vi "SolveIntersectionStrip.vi"(7 "ct":dbl=10.0 format="%.2f", 8 "Root method":bool, 10 "strip":cluster{"radius":dbl, "h":dbl, "w":dbl}={"radius"=10.0, "h"=5.0, "w"=4.0} {"radius" format="%.2f"; "w" format="%.2f"; "h" format="%.2f"}, 11 "P":cluster{"x":dbl, "y":dbl, "z":dbl}={"x"=-4.0, "y"=0.0, "z"=4.0} {"x" format="%.2f"; "z" format="%.2f"; "y" format="%.2f"}) -> (0 "XY Graph":T1(graph), 1 "Array":dbl[][](array[numeric]) format="%.2f", 2 "sigma":dbl=4.0 format="%.2f", 3 "d":dbl=4.0 format="%.2f")   [LabVIEW 2022 SP3]
uses:
  <vilib>/gmath/NI_Gmath.lvlib
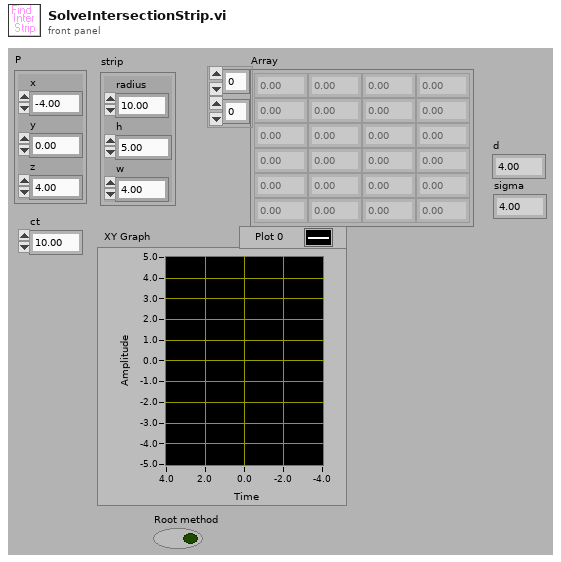
[diagram p1: front panel]
types:
  T1 = cluster{"Array Constant":dbl[], "Array Constant":dbl[]}[]
  T2 = cluster{"x,y,z[0]":dbl, "x,y,z[1]":dbl, "x,y,z[2]":dbl}
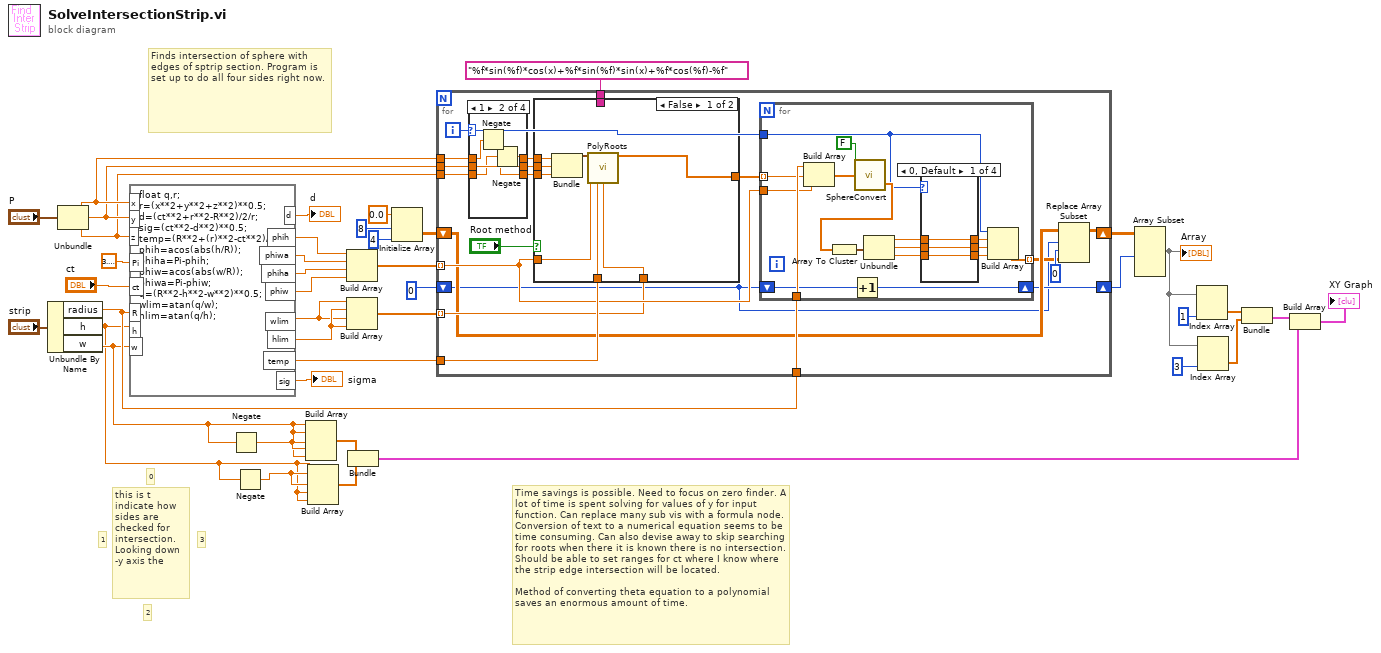
[diagram p0: block diagram]
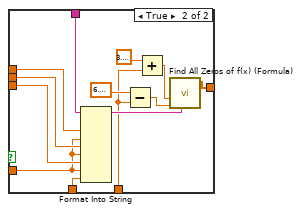
[diagram p2: hidden frame]
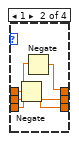
[diagram p3: hidden frame]
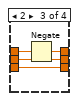
[diagram p4: hidden frame]
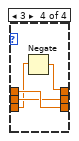
[diagram p5: hidden frame]
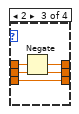
[diagram p7: hidden frame]
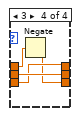
[diagram p8: hidden frame]
diagram:
  # "Finds intersection of sphere with edges of sptrip section. Program is set up to do all four sides right now."
  # "Time savings is possible. Need to focus on zero finder. A lot of time is spent solving for values of y for input function. Can replace many sub vis with a formula node. Conversion of text to a numerical equation seems to be time consuming. Can also devise away to skip searching for roots when there it is known there is no intersection. Should be able to set ranges for ct where I know where the strip edge intersection will be located.\n\nMethod of converting theta equation to a polynomial saves an enormous amount of time."
  # "3"
  # "2"
  # "1"
  # "0"
  # "this is t indicate how  sides are checked for intersection. Looking down -y axis the"
  n1 = Unbundle By Name("strip") -> ("radius"=w34:dbl, "h"=w13:dbl, "w"=w14:dbl)
  n2 = Unbundle("P") -> ("x"=w7:dbl, "y"=w6:dbl, "z"=w5:dbl)
  n3 = formula code="float q,r;\nr=(x**2+y**2+z**2)**0.5;\nd=(ct**2+r**2-R**2)/2/r;\nsig=(ct**2-d**2)**0.5;\ntemp=(R**2+(r)**2-ct**2)/2/R;\nphih=acos(abs(h/R));\nphiha=Pi-phih;\nphiw=acos(abs(w/R));\nphiwa=Pi-phiw;\nq=(R**2-h**2-w**2)**0.5;\nwlim=atan(q/w);\nhlim=atan(q/h);"("x"=w7, "y"=w6, "z"=w5, "ct"="ct", "R"=w34, "h"=w13, "w"=w14, "Pi"=3.141592653589793) -> ("d"=→"d":dbl, "sig"=→"sigma":dbl, "temp"=w38:dbl, "phih"=w28:dbl, "phiw"=w27:dbl, "phiha"=w31:dbl, "phiwa"=w32:dbl, "hlim"=w26:dbl, "wlim"=w25:dbl)
  n4 = Negate(x=w14) -> (-x=w20:dbl)
  n5 = Negate(x=w13) -> (-x=w19:dbl)
  n6 = Build Array(w14, w14, w20, w20, w14) -> (w18:dbl[])
  n7 = Build Array(w13, w19, w19, w13, w13) -> (w17:dbl[])
  n8 = Build Array(w28, w32, w31, w27) -> (w36:dbl[])
  n9 = Build Array(w25, w26, w25, w26) -> (w30:dbl[])
  n10 = Bundle(w18, w17) -> (w15:cluster{dbl[], dbl[]})  [unwired: 1 out]
  n11 = Initialize Array(0.0, 8, 4) -> (w11:dbl[][])
  n12 = for {
    tunnel: w38 -> [w61]
    tunnel: "%f*sin(%f)*cos(x)+%f*sin(%f)*sin(x)+%f*cos(%f)-%f" ("formula") -> [w57]
    tunnel: w36 -> [w55] mode=indexing
    tunnel: w34 -> [w54]
    shift-right: [w51] -> w10
    shift-left: w11 -> [w46]
    tunnel: w30 -> [w53] mode=indexing
    shift-right: [w44] -> w8
    shift-left: 0 -> [w43]
    tunnel: w7 -> [w49]
    tunnel: w6 -> [w48]
    tunnel: w5 -> [w47]
    i -> [w56]
    n13 = case shown="1" w56 {
      tunnel: [w118 w119 w124 w130] -> w60
      tunnel: w49 -> [w118 w121 w127 w129]
      tunnel: [w117 w123 w126 w131] -> w59
      tunnel: w48 -> [w117 w123 w126 w131]
      tunnel: [w116 w120 w125 w128] -> w58
      tunnel: w47 -> [w116 w122 w125 w130]
      frame 0, Default {
      }
      frame 1 {
        n14 = Negate(x=w121) -> (-x=w120:dbl)
        n15 = Negate(x=w122) -> (-x=w119:dbl)
      }
      frame 2 {
        n16 = Negate(x=w127) -> (-x=w124:dbl)
      }
      frame 3 {
        n17 = Negate(x=w129) -> (-x=w128:dbl)
      }
    }
    n18 = case shown="False" "Root method" {
      tunnel: w61 -> [w66 w82]
      tunnel: w60 -> [w65 w81]
      tunnel: w59 -> [w64 w80]
      tunnel: w58 -> [w63 w79]
      tunnel: w57 -> [_ w78]
      tunnel: w55 -> [w69 w77]
      tunnel: w53 -> [w67 w71]
      tunnel: [w68 w70] -> w52
      frame False {
        n19 = Bundle("z"=w65, "y"=w64, "z"=w63) -> (w62:cluster{"z":dbl, "y":dbl, "z":dbl})  [unwired: 1 out]
        n20 = call "PolyRoots.vi"("P"=w62, "phi"=w69, "constant"=w66, "theta lim"=w67) -> ("Polynomial Roots"=w68:dbl[])  [unwired: 2 in, 9 out]
      }
      frame True {
        n21 = Format Into String(format string=w78, w81, w77, w80, w77, w79, w77, w82) -> (resulting string=w76:string)  [unwired: 2 in, 1 out]
        n22 = Subtract(x=6.283185307179586, y=w71) -> (x-y=w75:dbl)
        n23 = Add(x=3.141592653589793, y=w71) -> (x+y=w73:dbl)
        n24 = call <vilib>:"Find All Zeros of f(x) (Formula).vi"("formula"=w76, "end"=w75, "start"=w73) -> ("Zeros"=w70:dbl[])  [unwired: 5 in, 3 out]
      }
    }
    n25 = for {
      tunnel: w52 -> [w98] mode=indexing
      tunnel: w56 -> [w85]
      tunnel: w54 -> [w99]
      tunnel: w55 -> [w97]
      tunnel: [w86] -> w45 mode=indexing
      shift-right: [w83] -> w44
      shift-left: w43 -> [w84]
      n26 = Build Array(w99, w98, w97) -> (w96:dbl[])
      n27 = Increment(x=w84) -> (x+1=w83:i32)
      n28 = call "SphereConvert.vi"("spherical in"=w96, "xyz ?"=FALSE) -> ("x,y,z"=w94:dbl[])  [unwired: 1 in, 1 out]
      n29 = Array To Cluster(array=w94) -> (cluster=w93:T2)
      n30 = Unbundle(w93) -> ("x,y,z[0]"=w92:dbl, "x,y,z[1]"=w91:dbl, "x,y,z[2]"=w90:dbl)
      n31 = case shown="0, Default" w85 {
        tunnel: [w102 w104 w108 w112] -> w89
        tunnel: w92 -> [w102 w107 w111 w115]
        tunnel: [w101 w106 w110 w114] -> w88
        tunnel: w91 -> [w101 w106 w110 w114]
        tunnel: [w100 w103 w109 w115] -> w87
        tunnel: w90 -> [w100 w105 w109 w113]
        frame 0, Default {
        }
        frame 1 {
          n32 = Negate(x=w107) -> (-x=w103:dbl)
          n33 = Negate(x=w105) -> (-x=w104:dbl)
        }
        frame 2 {
          n34 = Negate(x=w111) -> (-x=w108:dbl)
        }
        frame 3 {
          n35 = Negate(x=w113) -> (-x=w112:dbl)
        }
      }
      n36 = Build Array(w85, w89, w88, w87) -> (w86:dbl[])
    }
    n37 = Replace Array Subset(array=w46, new element=w45, index (row)=w43, index (col)=0) -> (w51:dbl[][])
  }
  n38 = Array Subset(array=w10, length (row)=w8) -> (w9:dbl[][])  [unwired: 3 in]
  "Array" <- w9
  n39 = Index Array(array=w9, index (col)=1) -> (element=w22:dbl[])  [unwired: 1 in]
  n40 = Index Array(array=w9, index (col)=3) -> (element=w21:dbl[])  [unwired: 1 in]
  n41 = Bundle(w22, w21) -> (w16:cluster{dbl[], dbl[]})  [unwired: 1 out]
  n42 = Build Array(w16, w15) -> (→"XY Graph":cluster{dbl[], dbl[]}[])
